vi "End Arduino Comms.vi"() -> (0 "Error":errorcluster)   [LabVIEW 2012]
uses:
  Arduino_comms_Global.vi
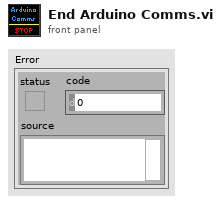
[diagram p1: front panel]
types:
  T1 = typedef "Arduino_comm_params.ctl" = cluster{"VISA resource name":refnum<visa-resource-name>, "byte count":u32, "flow control (0:none)":u16, "stop bits (10: 1 bit)":u16, "parity (0:none)":enum16{"None", "Odd", "Even", "Mark", "Space"}, "data bits (8)":u16, "termination char ":u8, "Enable Termination\nChar":bool, "baud rate (bps)":u32, "timeout (ms)":u32, "Locked":bool}
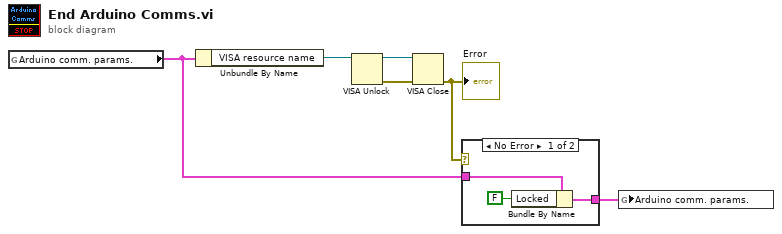
[diagram p0: block diagram]
diagram:
  n1 = global read "Arduino_comms_Global.vi" "Arduino comm. params."() -> (w2:T1)
  n2 = Unbundle By Name(w2) -> ("VISA resource name"=w4:refnum<visa-resource-name>)
  n3 = VISA Unlock(11:w4) -> (0:w6:errorcluster, 3:w5:refnum<visa-resource-name>)  [unwired: 1 in]
  n4 = VISA Close(VISA resource name=w5, error in (no error)=w6) -> (error out=w3:errorcluster)
  "Error" <- w3
  n5 = case shown="No Error" w3 {
    tunnel: [w7 w10] -> w1
    tunnel: w2 -> [w8 w10]
    frame No Error {
      n6 = Bundle By Name(cluster=w8, "Locked"=FALSE) -> (w7:T1)
    }
    frame Error {
    }
  }
  n7 = global write "Arduino_comms_Global.vi" "Arduino comm. params."(w1) -> ()
